vi "Get-Set 1D Fit Parameters.vi"(6 "Get(F)/Set":bool, 8 "Error In":errorcluster, 9 "Fixed Parameters":T7, 11 "Fit Settings":T1={"Use Original Plot # Points"=FALSE, "# Fit Plot Points"=0, "Fitting Method"=enum."Least Square", "Weighted Fit"=enum."Unweighted", "Show All Fit Components"=FALSE, "Axis Type"=0, "Show Fit Residuals"=TRUE, "Residual Type"=enum."Standard", "Fitting Algorithm"=enum."Levenberg-Marquardt", "Show Confidence Interval"=FALSE, "Confidence Level"=95.0} {"Confidence Level" min=0.0 max=100.0; "Axis Type" items=["Linear", "Logarithmic"]}) -> (0 "Error Out":errorcluster, 1 "Fixed Parameters":T7, 3 "Fit Settings":T1={"Use Original Plot # Points"=FALSE, "# Fit Plot Points"=0, "Fitting Method"=enum."Least Square", "Weighted Fit"=enum."Unweighted", "Show All Fit Components"=FALSE, "Axis Type"=0, "Show Fit Residuals"=TRUE, "Residual Type"=enum."Standard", "Fitting Algorithm"=enum."Levenberg-Marquardt", "Show Confidence Interval"=FALSE, "Confidence Level"=95.0} {"Confidence Level" min=0.0 max=100.0; "Axis Type" items=["Linear", "Logarithmic"]}, 4 "Initialized?":bool)   [LabVIEW 2021, in "Fits.lvlib"]
uses:
  Fits.lvlib
  D-Only Fixed Parameters.ctl
  Fit Settings.ctl
  Nonlinear Fit Method.ctl
  Ramp Type.ctl
  Residual Type.ctl
  Non-linear Fitting Algorithm.ctl
  IRF(X)PSED/Fit Weights Type v2.ctl
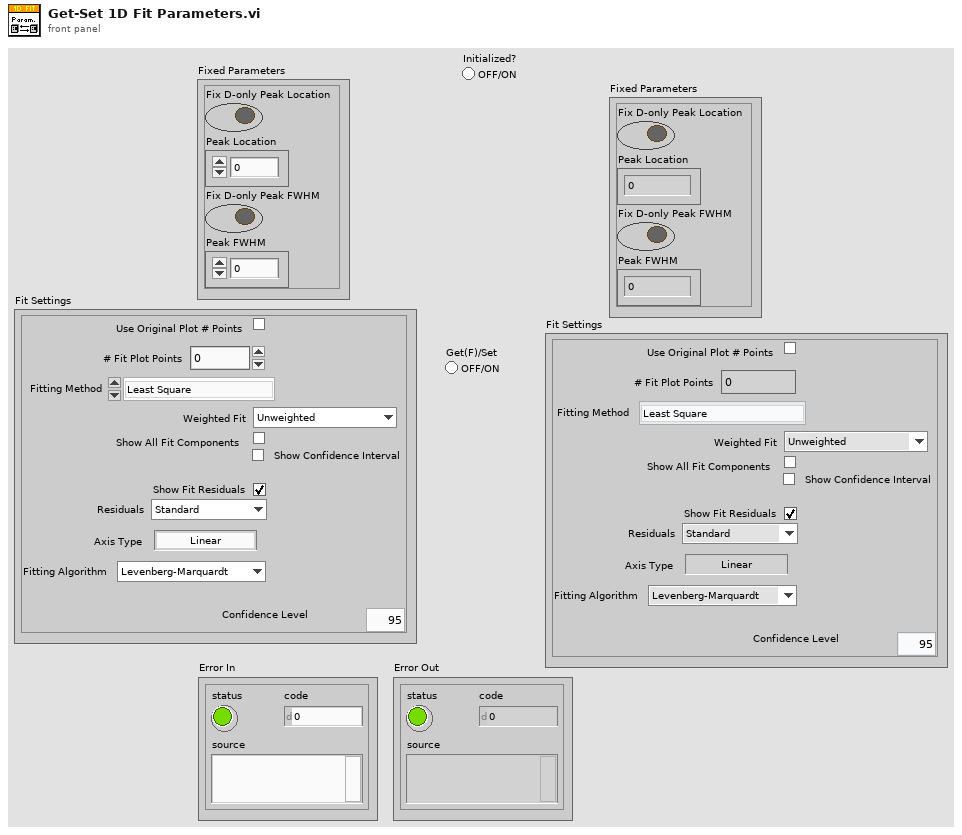
[diagram p1: front panel]
types:
  T1 = typedef "Fits.lvlib/Fit Settings.ctl" = cluster{"Use Original Plot # Points":bool, "# Fit Plot Points":u32, "Fitting Method":T2, "Weighted Fit":T3, "Show All Fit Components":bool, "Axis Type":T4, "Show Fit Residuals":bool, "Residual Type":T5, "Fitting Algorithm":T6, "Show Confidence Interval":bool, "Confidence Level":dbl}
  T2 = typedef "Fits.lvlib/Nonlinear Fit Method.ctl" = enum16{"Least Square", "Least Absolute Residual", "Bisquare", "MLE"}
  T3 = typedef "Fits.lvlib/Fit Weights Type v2.ctl" = enum16{"Unweighted", "1/Variance (Neyman)", "1/Variance (Pearson)", "Best of All"}
  T4 = typedef "Fits.lvlib/Ramp Type.ctl" = u16
  T5 = typedef "Fits.lvlib/Residual Type.ctl" = enum16{"Standard", "Normalized", "Reduced"}
  T6 = typedef "Fits.lvlib/Non-linear Fitting Algorithm.ctl" = enum16{"Levenberg-Marquardt", "Trust-Region Dogleg"}
  T7 = typedef "Fits.lvlib/D-Only Fixed Parameters.ctl" = cluster{"Fix D-only Peak Location":bool, "Peak Location":dbl, "Fix D-only Peak FWHM":bool, "Peak FWHM":dbl}
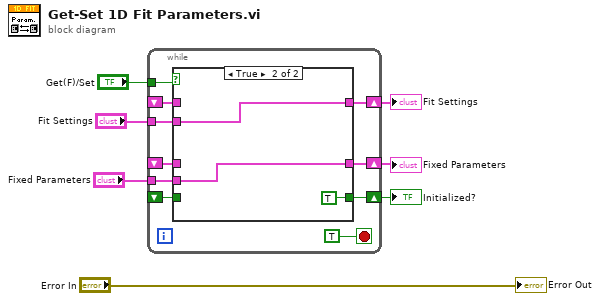
[diagram p0: block diagram]
diagram:
  n1 = while {
    tunnel: "Get(F)/Set" -> [w16]
    shift-right: [w14] -> w4
    shift-left: _ -> [w11]
    shift-right: [w13] -> w2
    shift-left: _ -> [w10]
    tunnel: "Fit Settings" -> [w15]
    tunnel: "Fixed Parameters" -> [w12]
    shift-right: [w9] -> w1
    shift-left: _ -> [w8]
    stop <- TRUE stop-if-true
    n2 = case shown="True" w16 {
      tunnel: w15 -> [_ w23]
      tunnel: [w20 w23] -> w14
      tunnel: [w19 w22] -> w13
      tunnel: w12 -> [_ w22]
      tunnel: w11 -> [w20 _]
      tunnel: w10 -> [w19 _]
      tunnel: [w18 TRUE] -> w9
      tunnel: w8 -> [w18 _]
      frame False {
      }
      frame True {
      }
    }
  }
  "Fixed Parameters" <- w2
  "Fit Settings" <- w4
  "Initialized?" <- w1
  "Error Out" <- "Error In"
